vi "UsrProfiles-Prevent manual changes.vi"(9 "Changes array ctrl (Old value)":T1[](array[typedef]), 10 "Changes array ctrl":refnum<vi>, 11 "Changes array ctrl (New value)":T1[](array[typedef])) -> (0 "error out":errorcluster)   [LabVIEW 2017]
uses:
  Typedefs/Changed parameter cluster.ctl
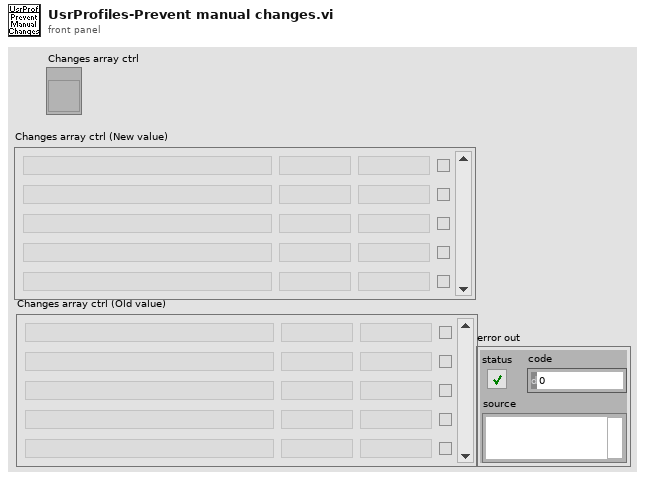
[diagram p1: front panel]
types:
  T1 = typedef "Changed parameter cluster.ctl" = cluster{"Name":string, "Old value":string, "New value":string, "Save":bool}
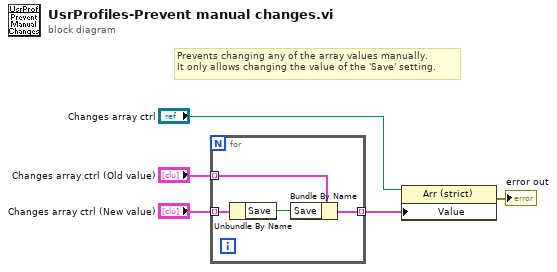
[diagram p0: block diagram]
diagram:
  # "Prevents changing any of the array values manually.\nIt only allows changing the value of the 'Save' setting."
  n1 = for {
    tunnel: "Changes array ctrl (Old value)" -> [w9] mode=indexing
    tunnel: "Changes array ctrl (New value)" -> [w8] mode=indexing
    tunnel: [w6] -> w3 mode=indexing
    n2 = Unbundle By Name(w8) -> ("Save"=w7:bool)
    n3 = Bundle By Name(cluster=w9, "Save"=w7) -> (w6:T1)
  }
  n4 = property class="Arr (strict)"(reference="Changes array ctrl", "Value"=w3) -> (error out=→"error out":errorcluster)  [unwired: 1 in, 1 out]
